vi "create_data_object.vi"(10 "Packet Size":i32=5000 caption="Numeric", 11 "data size":i32) -> (2 "data bus":T1, 3 "Test Data":T2)   [LabVIEW 2024, in "IPE Optimization Tester.lvlib"]
uses:
  IPE Optimization Tester.lvlib
  Tests/test_data--cluster.ctl
  data_bus--cluster.ctl
  <userlib>/_OpenG.lib/string/string.llb/openg_string.lvlib
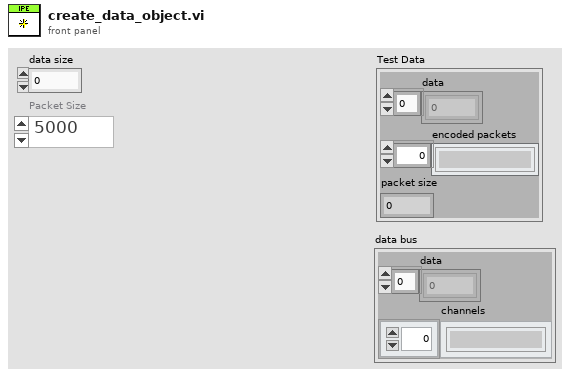
[diagram p1: front panel]
types:
  T1 = typedef "IPE Optimization Tester.lvlib/data_bus--cluster.ctl" = cluster{"data":dbl[], "channels":string[]}
  T2 = typedef "IPE Optimization Tester.lvlib/test_data--cluster.ctl" = cluster{"data":dbl[], "encoded packets":string[], "packet size":i32}
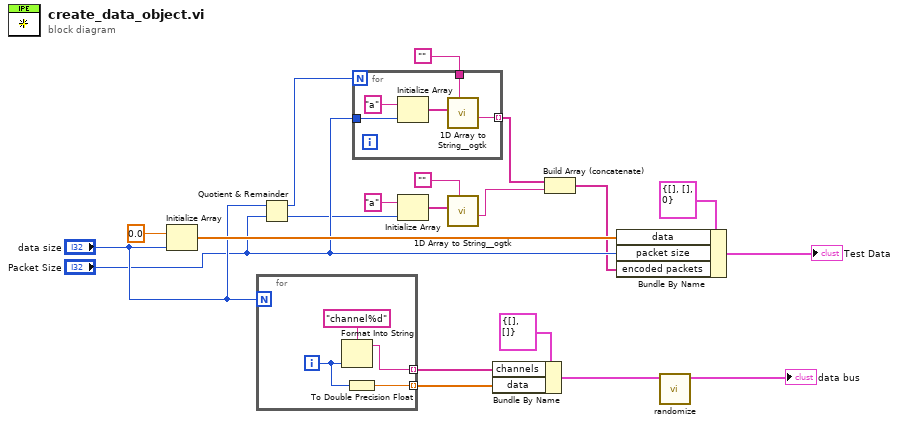
[diagram p0: block diagram]
diagram:
  n1 = Initialize Array(0.0, "data size") -> (w17:dbl[])
  n2 = for {
    N: "data size" -> [_]
    tunnel: [w22] -> w16 mode=indexing
    tunnel: [w21] -> w15 mode=indexing
    i -> [w23]
    n3 = Format Into String(format string="channel%d", w23) -> (resulting string=w21:string)  [unwired: 2 in, 1 out]
    n4 = To Double Precision Float(number=w23) -> (double precision float=w22:dbl)
  }
  n5 = Quotient & Remainder(x="data size", y="Packet Size") -> (x-y*floor(x/y)=w10:i32, floor(x/y)=w5:i32)
  n6 = for {
    N: w10 -> [_]
    tunnel: "Packet Size" -> [w29]
    tunnel: "" -> [w26]
    tunnel: [w25] -> w3 mode=indexing
    n7 = Initialize Array("a", w29) -> (w27:string[])
    n8 = call <userlib>:"1D Array to String__ogtk.vi"("delimiter (Tab)"=w26, "Array of Strings"=w27) -> ("delimited string"=w25:string)  [unwired: 9 in]
  }
  n9 = Initialize Array("a", w5) -> (w7:string[])
  n10 = call <userlib>:"1D Array to String__ogtk.vi"("delimiter (Tab)"="", "Array of Strings"=w7) -> ("delimited string"=w2:string)  [unwired: 9 in]
  n11 = Bundle By Name(cluster=T1 {"data"=[], "channels"=[]} ("packetized data"), "channels"=w15, "data"=w16) -> (w14:T1)
  n12 = Build Array (concatenate)(w3, w2) -> (w1:string[])
  n13 = Bundle By Name(cluster=T2 {"data"=[], "encoded packets"=[], "packet size"=0} ("test data"), "data"=w17, "packet size"="Packet Size", "encoded packets"=w1) -> (→"Test Data":T2)
  n14 = call "randomize.vi"("data bus"=w14) -> ("data bus out"=→"data bus":T1)  [unwired: 10 in]
